vi "FG_Camera.vi"(8 "Error":errorcluster, 10 "Camera Address":string="192.168.0.90", 11 "Action":T2) -> (0 "Error Out":errorcluster, 3 "CameraDevRef Out":T1, 5 "Camera Addresses":string[](array[string]))   [LabVIEW 2017, in "VisionSystem.lvlib"]
doc: "This software is licensed. Open the labview\\readme\\WPI Robotics Library Open Source License.txt file for more information."
uses:
  VisionSystem.lvlib
  <vilib>/Rock Robotics/WPI/Camera/WPI_CameraRegistryActions.ctl
  <vilib>/Rock Robotics/WPI/Camera/WPI_CameraDevRef.ctl
  <vilib>/Rock Robotics/WPI/Camera/WPI_CameraSettings Operations.ctl
  <vilib>/Rock Robotics/SystemInterfaces/NetworkCommunication/NetComm_UsageReport_ResourceType.ctl
  <vilib>/vision/driver/NI_Vision_Acquisition_Software.lvlib
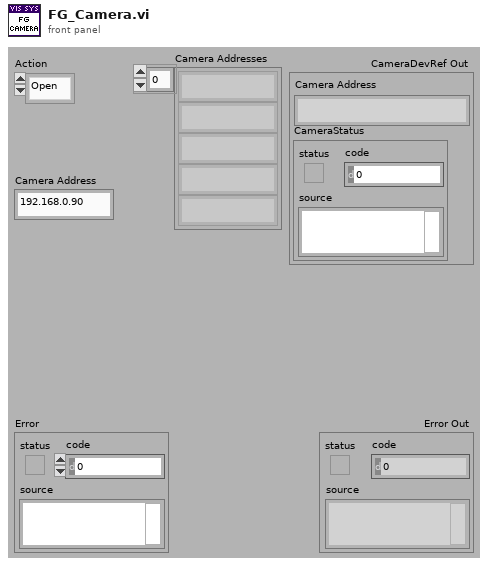
[diagram p1: front panel]
types:
  T1 = typedef "WPI_CameraDevRef.ctl" = cluster{"Camera Address":string, "CameraStatus":errorcluster}
  T2 = typedef "WPI_CameraRegistryActions.ctl" = enum16{"Open", "Close"}
  T3 = typedef "WPI_CameraSettings Operations.ctl" = enum16{"Udate FPS", "Update Compression", "Update Size", "Update White Balance", "Update Brightness", "Update Sharpness", "Update Exposure", "Update Exposure Value", "Update Color Level", "Update Exp Priority", "Update Color Enable", "Update JPG", "Update MJPG", "Read and Clear", "Read", "Init"}
  T4 = typedef "NetComm_UsageReport_ResourceType.ctl" = enum8{"Controller", "Module", "Language", "CANPlugin", "Accelerometer", "ADXL345", "AnalogChannel", "AnalogTrigger", "AnalogTriggerOutput", "CANJaguar", "Compressor", "Counter", "Dashboard", "DigitalInput", "DigitalOutput", "DriverStationCIO", "DriverStationEIO", "DriverStationLCD", "Encoder", "GearTooth", "Gyro", "I2C", "Framework", "Jaguar", "Joystick", "Kinect", "KinectStick", "PIDController", "Preferences", "PWM", "Relay", "RobotDrive", "SerialPort", "Servo", "Solenoid", "SPI", "Task", "Ultrasonic", "Victor", "Button", "Command", "AxisCamera", "PCVideoServer", "SmartDashboard", "Talon", "HiTechnicColorSensor", "HiTechnicAccel", "HiTechnicCompass", "SRF08", "AnalogOutput", "Victor SP", "Talon SRX", "CAN Talon SRX", "ADXL362 Accel", "ADXRS450 Gyro", "Rev SPARK", "Mindsensors SD540", "Digital Filter", "ADIS16448", "PDP", "PCM", "PigeonIMU", "Nidec Brushless", "CTRE CANifier", "CTRE Future 0", "CTRE Future 1", "CTRE Future 2", "CTRE Future 3", "CTRE Future 4", "CTRE Future 5", "CTRE Future 6"}
  T5 = typedef "WPI_CameraSettings Control.ctl" = cluster{"FPS":i32, "Compression":i32, "Size":i32, "White Balance":i32, "Brightness":i32, "Sharpness":i32, "Exposure":i32, "Color Level":i32, "Exposure Priority":i32, "Color Enable":i32, "JPG Loop":i32, "MJPG Loop":i32, "Exposure Value":i32}
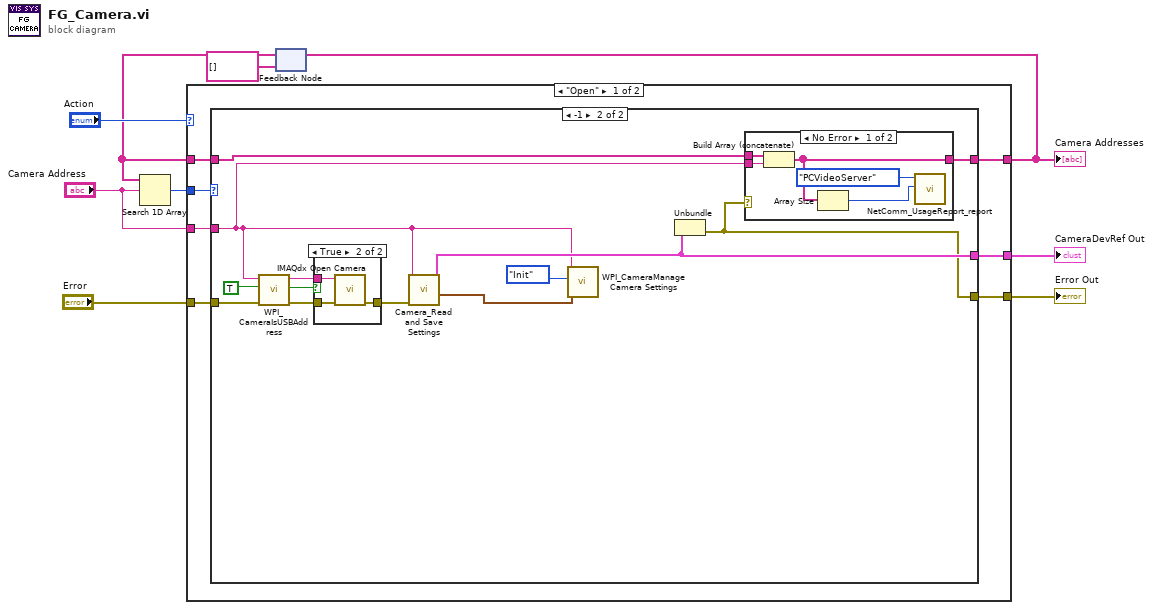
[diagram p0: block diagram]
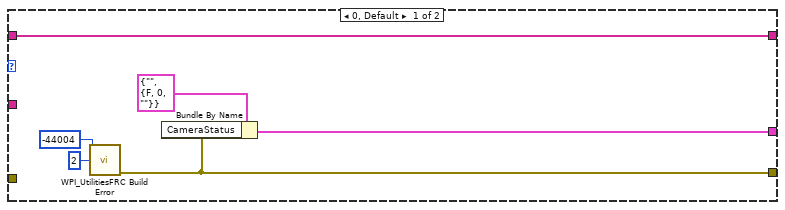
[diagram p2: hidden frame]
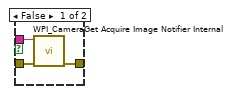
[diagram p3: hidden frame]
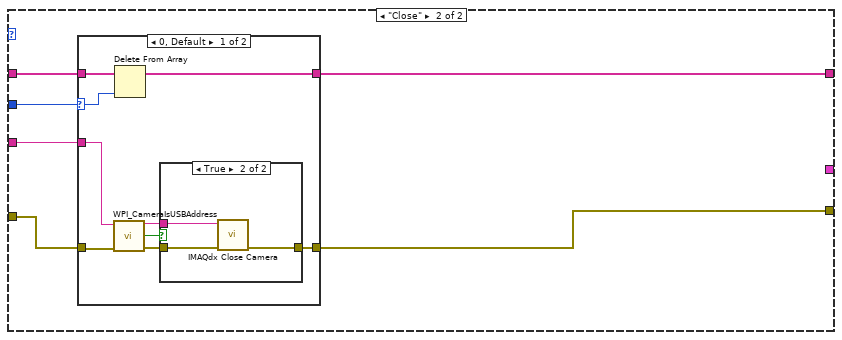
[diagram p5: hidden frame]
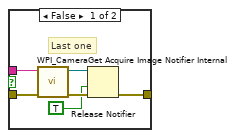
[diagram p6: hidden frame]
diagram:
  n1 = feedback #1(string[] []) -> (w3:string[])
  n2 = Search 1D Array(1D array=w3, element="Camera Address") -> (index of element=w4:i32)  [unwired: 1 out]
  n3 = case shown="\"Open\"" "Action" {
    tunnel: w3 -> [w15 w52]
    tunnel: "Camera Address" -> [w16 w48]
    tunnel: [w14 _] -> w8
    tunnel: w4 -> [w13 w53]
    tunnel: [w12 w51] -> w5
    tunnel: "Error" -> [w11 w50]
    tunnel: [w10 w49] -> w6
    frame "Open" {
      n4 = case shown="-1" w13 {
        tunnel: w16 -> [_ w25]
        tunnel: w15 -> [w22 w35]
        tunnel: [w21 w27] -> w14
        tunnel: [w22 w34] -> w12
        tunnel: w11 -> [_ w32]
        tunnel: [w18 w26] -> w10
        frame 0, Default {
          n5 = call <vilib>:"WPI_UtilitiesFRC Build Error.vi"("error code"=-44004 ("code"), "chain levels to remove (1)"=2) -> ("error out"=w18:errorcluster)  [unwired: 3 in, 10 out]
          n6 = Bundle By Name(cluster=T1 {"Camera Address"="", "CameraStatus"={"status"=FALSE, "code"=0, "source"=""}} ("CameraDevRef"), "CameraStatus"=w18) -> (w21:T1)
        }
        frame -1 {
          n7 = call <vilib>:"WPI_CameraIsUSBAddress.vi"("error in (no error)"=w32, "Enumerate?"=TRUE, "Camera Address In"=w25) -> ("error out"=w31:errorcluster, "USB?"=w29:bool, "Camera Address Out"=w30:string)  [unwired: 6 in]
          n8 = case shown="True" w29 {
            tunnel: [w38 w40] -> w33
            tunnel: w31 -> [w37 w41]
            tunnel: w30 -> [w36 w39]
            frame False {
              n9 = call <vilib>:"WPI_CameraGet Acquire Image Notifier Internal.vi"("error in (no error)"=w37, "Camera Address"=w36) -> ("error out"=w38:errorcluster)  [unwired: 9 out]
            }
            frame True {
              n10 = call <vilib>:"IMAQdx Open Camera.vi"("error in"=w41, "Session In"=w39) -> ("error out"=w40:errorcluster)  [unwired: 8 in, 1 out]
            }
          }
          n11 = call "Camera_Read and Save Settings.vi"("Error"=w33, "Camera Address"=w25) -> ("Output Cluster Out"=w23:T5, "CameraDevRef Out"=w27:T1)  [unwired: 6 in, 2 out]
          n12 = call <vilib>:"WPI_CameraManage Camera Settings.vi"("Values In"=w23, "Operation"=WPI_CameraSettings_Operations."Init", "Camera IP"=w25) -> ()  [unwired: 7 in, 2 out]
          n13 = Unbundle(w27) -> ("CameraStatus"=w26:errorcluster)  [unwired: 1 out]
          n14 = case shown="No Error" w26 {
            tunnel: w35 -> [w46 w47]
            tunnel: w25 -> [w45 _]
            tunnel: [w43 w47] -> w34
            frame No Error {
              n15 = Build Array (concatenate)(w46, w45) -> (w43:string[])
              n16 = Array Size(array=w43) -> (size(s)=w42:i32)
              n17 = call <vilib>:"NetComm_UsageReport_report.vi"("Instance Number"=w42, "Resource Type"=NetComm_UsageReport_ResourceType."PCVideoServer") -> ()  [unwired: 10 in]
            }
            frame Error {
            }
          }
        }
      }
    }
    frame "Close" {
      n18 = case shown="0, Default" w53 {
        selector: w53 -> [w59 _]
        tunnel: w52 -> [w62 w73]
        tunnel: [w61 w73] -> w51
        tunnel: w50 -> [w57 w72]
        tunnel: [w60 w72] -> w49
        tunnel: w48 -> [w56 _]
        frame 0, Default {
          n19 = call <vilib>:"WPI_CameraIsUSBAddress.vi"("error in (no error)"=w57, "Camera Address In"=w56) -> ("error out"=w58:errorcluster, "USB?"=w54:bool, "Camera Address Out"=w55:string)  [unwired: 7 in]
          n20 = Delete From Array(array=w62, index=w59) -> (array with subset deleted=w61:string[])  [unwired: 1 in, 1 out]
          n21 = case shown="True" w54 {
            tunnel: w58 -> [w68 w70]
            tunnel: [w67 w69] -> w60
            tunnel: w55 -> [w63 w71]
            frame False {
              # "Last one"
              n22 = call <vilib>:"WPI_CameraGet Acquire Image Notifier Internal.vi"("error in (no error)"=w68, "Camera Address"=w63) -> ("error out"=w66:errorcluster, "Acquire Image Notifier"=w65:refnum<notifier>)  [unwired: 8 out]
              n23 = Release Notifier(notifier=w65, force destroy? (F)=TRUE, error in (no error)=w66) -> (error out=w67:errorcluster)  [unwired: 2 out]
            }
            frame True {
              n24 = call <vilib>:"IMAQdx Close Camera.vi"("error in"=w70, "Session In"=w71) -> ("error out"=w69:errorcluster)  [unwired: 9 in]
            }
          }
        }
        frame -1 {
        }
      }
    }
  }
  "CameraDevRef Out" <- w8
  "Error Out" <- w6
  "Camera Addresses" <- w5
  n25 = feedback-in #1(w5) -> ()
